vi "Remote Time Check.vi"(7 "Tolerance (2 ms)":u32=2, 8 "error in (no error)":errorcluster, 9 "Number of Attempts (5)":u32=5, 10 "remote port (1234)":u16=1234, 11 "address (localhost)":string="localhost") -> (0 "error out":errorcluster, 1 "Windows OS Up Time (ms)":u32, 2 "Remote OS Up Time (ms)":u32)   [LabVIEW 2010, in "Core SubVIs.lvlib"]
doc: "Checks the OS Up Time of a remote computer over a TCP connection."
uses:
  Core SubVIs.lvlib
  TYPE - Remote Time Check State Control.ctl
panel:
  out "Number of Attempts":u32
  out "Valid Trip Time":bool
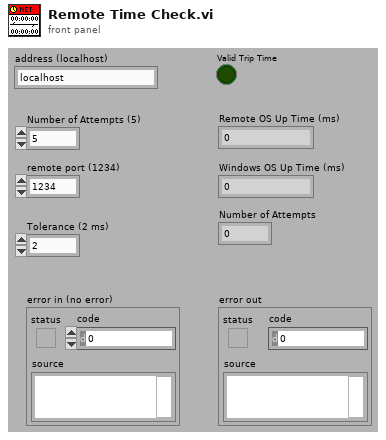
[diagram p1: front panel]
types:
  T1 = typedef "Core SubVIs.lvlib/TYPE - Remote Time Check State Control.ctl" = enum16{"Default", "Open Connection", "Check Time", "Close Connection", "Cleanup"}
  T2 = enum16{"Standard", "Buffered", "CRLF", "Immediate"}
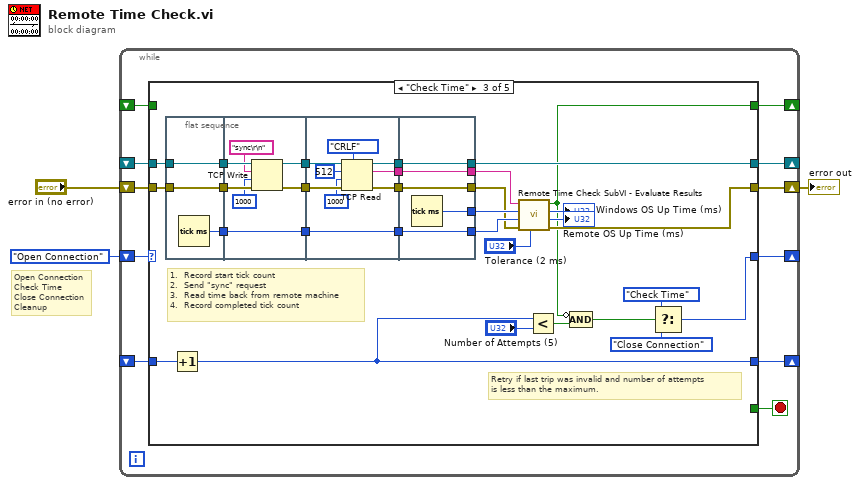
[diagram p0: block diagram]
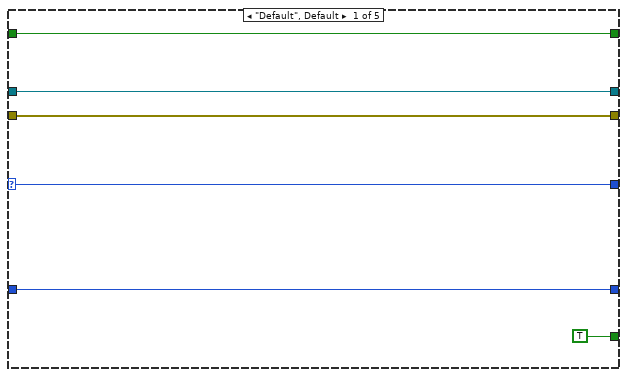
[diagram p2: hidden frame]
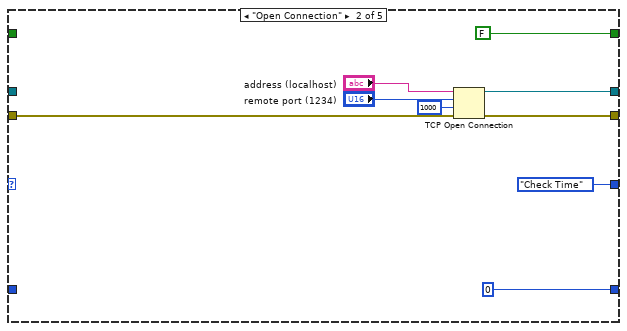
[diagram p3: hidden frame]
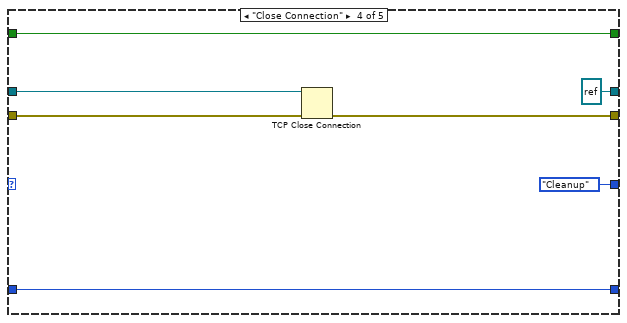
[diagram p4: hidden frame]
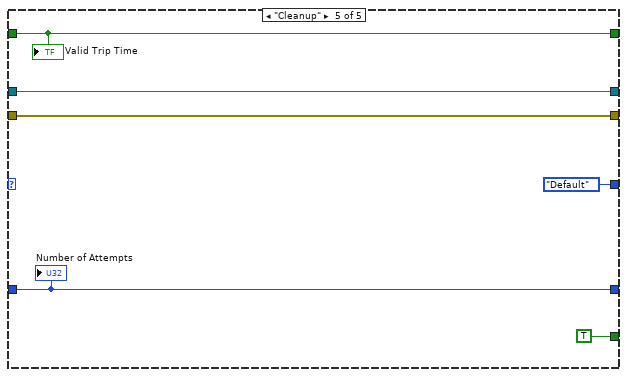
[diagram p5: hidden frame]
diagram:
  # "Open Connection\nCheck Time\nClose Connection\nCleanup"
  n1 = while {
    shift-right: [w13] -> _
    shift-left: TYPE_-_Remote_Time_Check_State_Control."Open Connection" ("State") -> [w14]
    shift-right: [w10] -> w1
    shift-left: "error in (no error)" -> [w9]
    shift-right: [w11] -> _
    shift-left: _ -> [w8]
    shift-right: [w7] -> _
    shift-left: _ -> [w6]
    shift-right: [w5] -> _
    shift-left: _ -> [w4]
    stop <- w12 stop-if-true
    n2 = case shown="\"Check Time\"" w14 {
      selector: w14 -> [w19 _ _ _ _]
      tunnel: [w19 TYPE_-_Remote_Time_Check_State_Control."Check Time" ("State") w31 TYPE_-_Remote_Time_Check_State_Control."Cleanup" ("State") TYPE_-_Remote_Time_Check_State_Control."Default" ("State")] -> w13
      tunnel: [TRUE _ _ _ TRUE] -> w12
      tunnel: [w16 w28 w47 refnum<k5> refnum ("connection ID") w96] -> w11
      tunnel: [w15 w27 w42 w87 w95] -> w10
      tunnel: w9 -> [w15 w23 w58 w88 w95]
      tunnel: w8 -> [w16 _ w59 w89 w96]
      tunnel: [w18 u32 0 w36 w84 w94] -> w7
      tunnel: w6 -> [w18 _ w38 w84 w94]
      tunnel: [w17 FALSE ("Valid Trip Time") w30 w90 w91] -> w5
      tunnel: w4 -> [w17 _ _ w90 w91]
      frame "Default", Default {
      }
      frame "Open Connection" {
        n3 = TCP Open Connection(address="address (localhost)", remote port or service name="remote port (1234)", timeout ms (60000)=1000, error in (no error)=w23) -> (connection ID=w28:refnum<k5>, error out=w27:errorcluster)  [unwired: 1 in]
      }
      frame "Check Time" {
        # "Retry if last trip was invalid and number of attempts\nis less than the maximum."
        # "1.  Record start tick count\n2.  Send \"sync\" request\n3.  Read time back from remote machine\n4.  Record completed tick count"
        n4 = flat-sequence {
          tunnel: w59 -> [w62]
          tunnel: w58 -> [w61]
          tunnel: [w62] -> w57
          tunnel: [w61] -> w56
          tunnel: [w60] -> w55
          tunnel: w57 -> [w69]
          tunnel: w56 -> [w66]
          tunnel: w55 -> [w68]
          tunnel: [w67] -> w54
          tunnel: [w68] -> w53
          tunnel: [w65] -> w52
          tunnel: w54 -> [w78]
          tunnel: w53 -> [w77]
          tunnel: w52 -> [w73]
          tunnel: [w76] -> w51
          tunnel: [w77] -> w50
          tunnel: [w71] -> w49
          tunnel: [w70] -> w48
          tunnel: [w80] -> w45
          tunnel: [w81] -> w43
          tunnel: [w82] -> w46
          tunnel: [w83] -> w47
          tunnel: w51 -> [w83]
          tunnel: w50 -> [w82]
          tunnel: w49 -> [w81]
          tunnel: w48 -> [w80]
          tunnel: [w79] -> w44
          frame #0 {
            n5 = Tick Count (ms)() -> (millisecond timer value=w60:u32)
          }
          frame #1 {
            n6 = TCP Write(connection ID=w69, data in="sync\r\n", error in (no error)=w66, 9:1000 ("timeout ms (25000)")) -> (connection ID out=w67:refnum<k5>, error out=w65:errorcluster)  [unwired: 1 out]
          }
          frame #2 {
            n7 = TCP Read(connection ID=w78, bytes to read=512, error in (no error)=w73, 7:T2."CRLF" ("mode (standard)"), 9:1000 ("timeout ms (25000)")) -> (connection ID out=w76:refnum<k5>, data out=w70:string, error out=w71:errorcluster)
          }
          frame #3 {
            n8 = Tick Count (ms)() -> (millisecond timer value=w79:u32)
          }
        }
        n9 = Increment(x=w38) -> (x+1=w36:u32)
        n10 = call "Remote Time Check SubVI - Evaluate Results.vi"("Tolerance (ms)"="Tolerance (2 ms)", "error in (no error)"=w43, "Start Tick Count (ms)"=w46, "Completion Tick Count (ms)"=w44, "Remote Time String (ms)"=w45) -> ("error out"=w42:errorcluster, "Remote OS Up Time (ms)"=→"Remote OS Up Time (ms)":u32, "Windows OS Up Time (ms)"=→"Windows OS Up Time (ms)":u32, "Valid Trip Time"=w30:bool)  [unwired: 3 in]
        n11 = Less?(x=w36, y="Number of Attempts (5)") -> (x < y?=w37:bool)
        n12 = Compound Arithmetic op=AND(invert w30, w37) -> (w34:bool)
        n13 = Select(t=TYPE_-_Remote_Time_Check_State_Control."Check Time" ("State"), s=w34, f=TYPE_-_Remote_Time_Check_State_Control."Close Connection" ("State")) -> (s? t:f=w31:T1)
      }
      frame "Close Connection" {
        n14 = TCP Close Connection(connection ID=w89, error in (no error)=w88) -> (error out=w87:errorcluster)  [unwired: 1 in, 1 out]
      }
      frame "Cleanup" {
        "Valid Trip Time" <- w91
        "Number of Attempts" <- w94
      }
    }
  }
  "error out" <- w1
